vi "Write Fault Event.vi"(8 "error in":errorcluster, 10 "Fault event":refnum<user-event>, 11 "Fault_Engine in":refnum<class "Engine.lvclass">) -> (0 "error out":errorcluster, 3 "Fault_Engine out":refnum<class "Engine.lvclass">)   [LabVIEW 2019, in "Engine.lvlib" / "Engine.lvclass"]
uses:
  Project/Engine.lvclass
  Project/Engine.lvclass/Engine.ctl
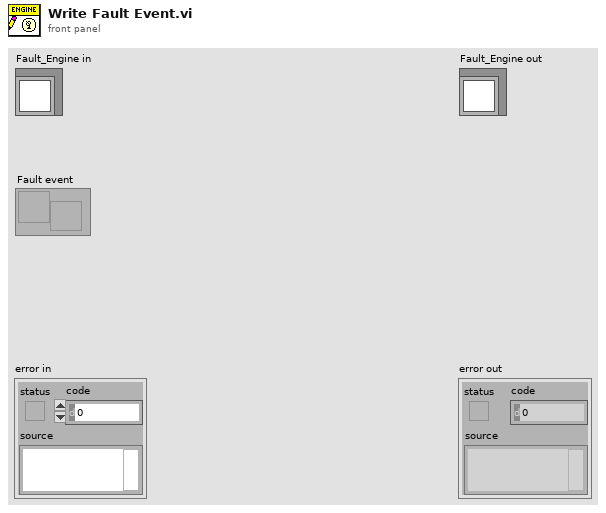
[diagram p1: front panel]
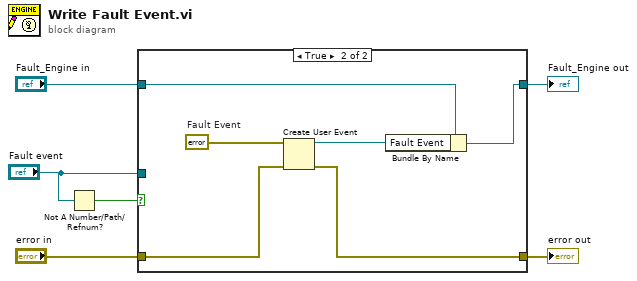
[diagram p0: block diagram]
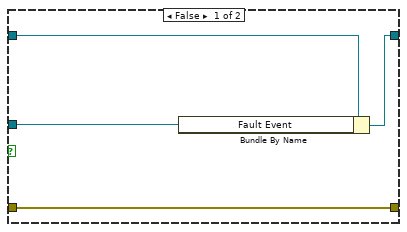
[diagram p2: hidden frame]
diagram:
  n1 = Not A Number/Path/Refnum?(number/path/refnum="Fault event") -> (NaN/Path/Refnum?=w3:bool)
  n2 = case shown="True" w3 {
    tunnel: [w7 w11] -> w6
    tunnel: [w9 w14] -> w4
    tunnel: "Fault_Engine in" -> [w10 w15]
    tunnel: "Fault event" -> [w8 _]
    tunnel: "error in" -> [w7 w12]
    frame False {
      n3 = Bundle By Name(cluster=w10, "Fault Event"=w8) -> (w9:refnum<class "Engine.lvclass">)
    }
    frame True {
      w16 = errorcluster {"status"=FALSE, "code"=0, "source"=""}  # Fault Event
      n4 = Create User Event(user event datatype=w16, error in=w12) -> (user event=w13:refnum<user-event>, error out=w11:errorcluster)
      n5 = Bundle By Name(cluster=w15, "Fault Event"=w13) -> (w14:refnum<class "Engine.lvclass">)
    }
  }
  "error out" <- w6
  "Fault_Engine out" <- w4
